vi "Diagnostic Data Lookup Table Initialize.vi"(8 "error in (no error)":errorcluster, 11 "Internal Command Engine References":T1 {"Command Refs"."Block Data Refs"."Data Reference" format="%.0x"; "Response Refs"."Block Data Refs" format="%.0x"}) -> (0 "error out":errorcluster {"code" min=0 max=0}, 3 "Diag Data Ref":T4)   [LabVIEW 2013, in "J1939 Addon Engine.lvlib"]
uses:
  J1939 Addon Engine.lvlib
  Types/Diagnostic Data Lookup Table Reference.ctl
  Types/Internal Command Configuration Parameters.ctl
  <vilib>/NI Veristand/Custom Device API/Data Reference.ctl
  <vilib>/NI Veristand/Custom Device API/Block Data Reference.ctl
  Types/Diagnostic Data Lookup Table Action.ctl
  <vilib>/NI Veristand/Custom Device API/Custom Device API.lvlib
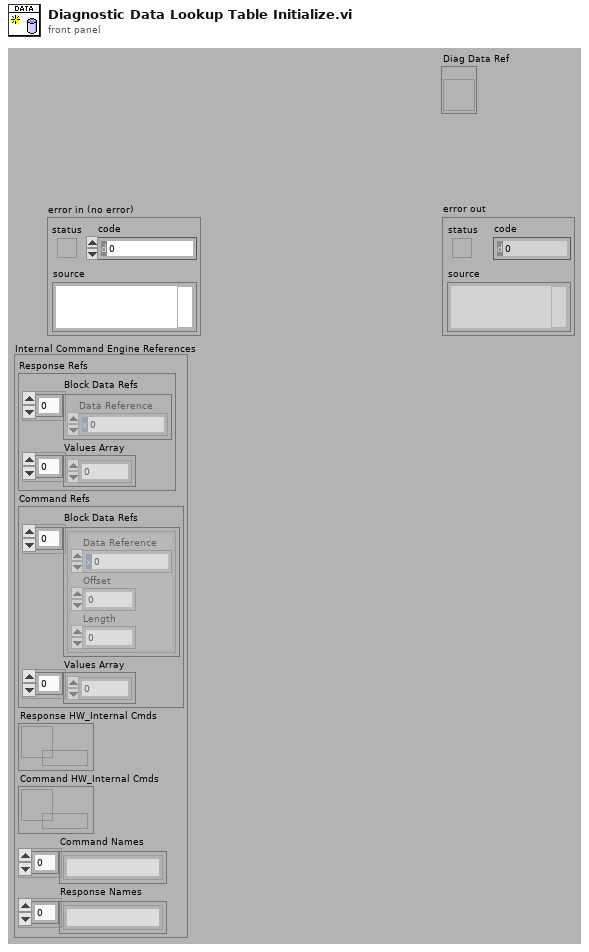
[diagram p1: front panel]
types:
  T1 = typedef "J1939 Addon Engine.lvlib/Internal Command Configuration Parameters.ctl" = cluster{"Response Refs":cluster{"Block Data Refs":T2[], "Values Array":dbl[]}, "Command Refs":cluster{"Block Data Refs":T3[], "Values Array":dbl[]}, "Response HW_Internal Cmds":refnum<k33>, "Command HW_Internal Cmds":refnum<k33>, "Command Names":string[], "Response Names":string[]}
  T2 = typedef "Custom Device API.lvlib/Data Reference.ctl" = i32
  T3 = typedef "Custom Device API.lvlib/Block Data Reference.ctl" = cluster{"Data Reference":T2, "Offset":i32, "Length":i32}
  T4 = typedef "J1939 Addon Engine.lvlib/Diagnostic Data Lookup Table Reference.ctl" = refnum<vi>
  T5 = typedef "J1939 Addon Engine.lvlib/Diagnostic Data Lookup Table Action.ctl" = enum16{"Initialize", "Get All", "Set All", "Set Value", "Get Value"}
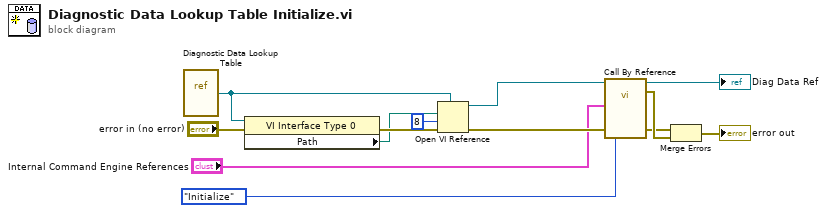
[diagram p0: block diagram]
diagram:
  n1 = vi-ref "Diagnostic Data Lookup Table.vi"() -> (w13:refnum<vi>)
  n2 = property class="VI Interface Type 0"(reference=w13, error in="error in (no error)") -> (error out=w11:errorcluster, "Path"=w4:path)  [unwired: 1 out]
  n3 = Open VI Reference(type specifier VI Refnum (for type only)=w13, vi path=w4, options=8, error in (no error)=w11) -> (vi reference=w10:refnum<vi>, error out=w6:errorcluster)  [unwired: 2 in]
  n4 = call-by-ref "?"(reference=w10, "command"=Diagnostic_Data_Lookup_Table_Action."Initialize", "error in (no error)"=w6, "Internal Command Engine References"="Internal Command Engine References") -> (reference out=→"Diag Data Ref":refnum<vi>, error out=w9:errorcluster, 0:"error out"=w5:errorcluster)  [unwired: 7 in, 2 out]
  n5 = Merge Errors(w5, w9) -> (→"error out":errorcluster)
